vi "Siemens ELAN CRC16 calculator.vi"(2 "CRC16 seed":u16=65535 format="%.0x", 3 "Input String":string) -> (0 "CRC16 output":u16 format="%.0x", 1 "String with CRC16":string)   [LabVIEW 2020, in "Siemens ELAN.lvlib"]
doc: "Calculates a 16-bit CRC of the input string as a byte sequence, using the supplied seed. Returns the CRC16 and also a copy of the string with the two-byte CRC appended, MSB first.\n\nCRC seed if unwired defaults to 0xFFFF. Seed and mask conform to the x^16 + x^15 + x^2 + 1 polynomial used by Siemens ELAN protocol."
uses:
  Siemens ELAN.lvlib
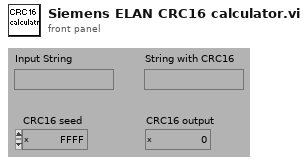
[diagram p1: front panel]
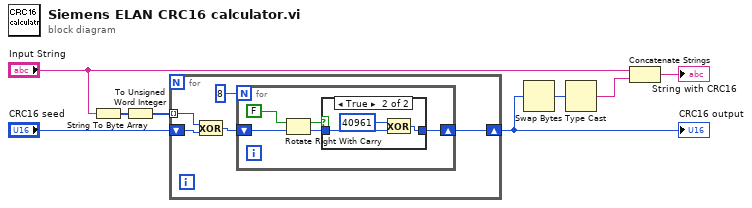
[diagram p0: block diagram]
diagram:
  n1 = String To Byte Array(string="Input String") -> (unsigned byte array=w8:u8[])
  n2 = To Unsigned Word Integer(number=w8) -> (unsigned 16bit integer=w3:u16[])
  n3 = for {
    shift-right: [w12] -> w2
    shift-left: "CRC16 seed" -> [w9]
    tunnel: w3 -> [w11] mode=indexing
    n4 = Exclusive Or(1:w9, 2:w11) -> (0:w10:u16)
    n5 = for {
      N: 8 -> [_]
      shift-right: [w18] -> w12
      shift-left: w10 -> [w14]
      n6 = Rotate Right With Carry(2:w14, 3:FALSE ("carry")) -> (0:w15:u16, 1:w16:bool)
      n7 = case shown="True" w16 {
        tunnel: w15 -> [w19 w20]
        tunnel: [w19 w22] -> w18
        frame False {
        }
        frame True {
          n8 = Exclusive Or(1:w20, 2:u16 40961) -> (0:w22:u16)
        }
      }
    }
  }
  "CRC16 output" <- w2
  n9 = Swap Bytes(anything=w2) -> (byte swapped=w1:u16)
  n10 = Type Cast(x=w1) -> (*(type *) &x=w4:string)  [unwired: 1 in]
  n11 = Concatenate Strings("Input String", w4) -> (→"String with CRC16":string)
